vi "CreateWaveformMatlabCoerced.vi"(10 "WaveDuration (us)":dbl=2e-05, 11 "Freq US  (Hz)":dbl=6000000.0) -> (0 "NCH1 high":i32=10, 1 "Freq CH1  (Hz)":dbl, 2 "Nlow":i32, 3 "Freq Low":dbl, 4 "NCH2 high":dbl, 5 "sampling frequency":dbl, 6 "Freq CH2 (Hz)":dbl)   [LabVIEW 2015]
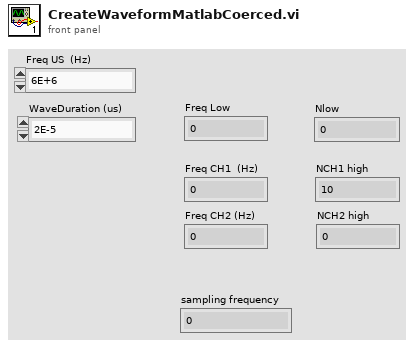
[diagram p1: front panel]
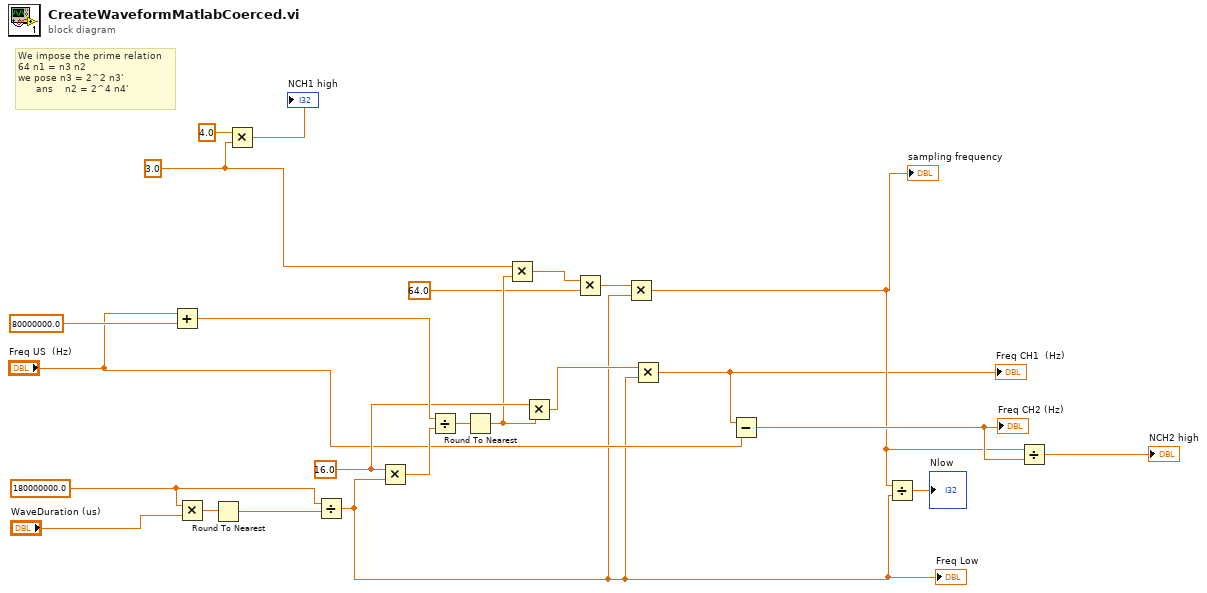
[diagram p0: block diagram]
diagram:
  w12 = 16.0 ("x")
  w9 = 3.0 ("x")
  w21 = 180000000.0 ("y")
  # "We impose the prime relation\n64 n1 = n3 n2\nwe pose n3 = 2^2 n3'\n      ans    n2 = 2^4 n4'"
  n1 = Add(x="Freq US  (Hz)", y=80000000.0 ("x")) -> (x+y=w14:dbl)
  n2 = Multiply(x=w21, y="WaveDuration (us)") -> (x*y=w23:dbl)
  n3 = Round To Nearest(number=w23) -> (nearest integer value=w20:dbl)
  n4 = Multiply(x=4.0, y=w9) -> (x*y=→"NCH1 high":dbl)
  n5 = Divide(x=w21, y=w20) -> (x/y=w3:dbl)
  "Freq Low" <- w3
  n6 = Multiply(x=w12, y=w3) -> (x*y=w15:dbl)
  n7 = Divide(x=w14, y=w15) -> (x/y=w13:dbl)
  n8 = Round To Nearest(number=w13) -> (nearest integer value=w10:dbl)
  n9 = Multiply(x=w9, y=w10) -> (x*y=w8:dbl)
  n10 = Multiply(x=w12, y=w10) -> (x*y=w11:dbl)
  n11 = Multiply(x=w8, y=64.0 ("x")) -> (x*y=w5:dbl)
  n12 = Multiply(x=w5, y=w3) -> (x*y=w6:dbl)
  "sampling frequency" <- w6
  n13 = Multiply(x=w11, y=w3) -> (x*y=w1:dbl)
  "Freq CH1  (Hz)" <- w1
  n14 = Subtract(x=w1, y="Freq US  (Hz)") -> (x-y=w18:dbl)
  "Freq CH2 (Hz)" <- w18
  n15 = Divide(x=w6, y=w3) -> (x/y=→"Nlow":dbl)
  n16 = Divide(x=w6, y=w18) -> (x/y=→"NCH2 high":dbl)
